vi "Get Process Model.vi"(8 "error in (no error)":errorcluster, 11 "Execution in":refnum<class "Execution.lvclass">) -> (0 "error out":errorcluster, 2 "Process Model":T1, 3 "Execution out":refnum<class "Execution.lvclass">)   [LabVIEW 2020, in "TSS.lvlib" / "Execution.lvclass"]
uses:
  Execution.lvclass
  SequenceFile/Typedefs/Session Handle.ctl
  SequenceFile/SequenceFile.lvclass
  Execution.lvclass/Execution.ctl
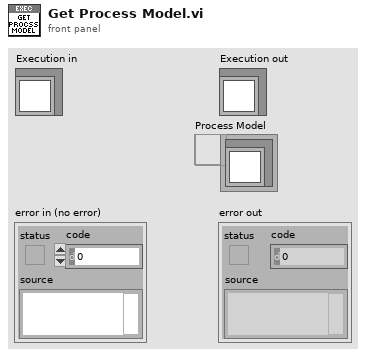
[diagram p1: front panel]
types:
  T1 = typedef "TSS.lvlib/SequenceFile.lvclass/Session Handle.ctl" = refnum<data-value>
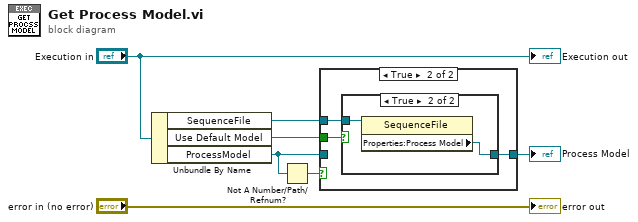
[diagram p0: block diagram]
diagram:
  n1 = Unbundle By Name("Execution in") -> ("SequenceFile"=w2:T1, "Use Default Model"=w4:bool, "ProcessModel"=w3:T1)
  n2 = Not A Number/Path/Refnum?(number/path/refnum=w3) -> (NaN/Path/Refnum?=w5:bool)
  n3 = case shown="True" w5 {
    tunnel: w4 -> [_ w11]
    tunnel: w3 -> [w8 _]
    tunnel: w2 -> [_ w10]
    tunnel: [w8 w9] -> w1
    frame False {
    }
    frame True {
      n4 = case shown="True" w11 {
        tunnel: w10 -> [_ w13]
        tunnel: [_ w12] -> w9
        frame False {
        }
        frame True {
          n5 = property class="SequenceFile"(reference=w13) -> ("Properties:Process Model"=w12:T1)  [unwired: 1 in, 2 out]
        }
      }
    }
  }
  "Process Model" <- w1
  "error out" <- "error in (no error)"
  "Execution out" <- "Execution in"
